vi "Scope Multi Point Read.vi"() -> ()   [LabVIEW 2013]
uses:
  Power Supply.lvlib
  Fixture.lvlib
  Oscilloscope.lvlib
panel:
  in  "outputVoltage":dbl=9.0 format="%#_13g"
  out "Waveform Graph":dbl[](graph)
  in  "Channel":i32=2
  out "error out":errorcluster
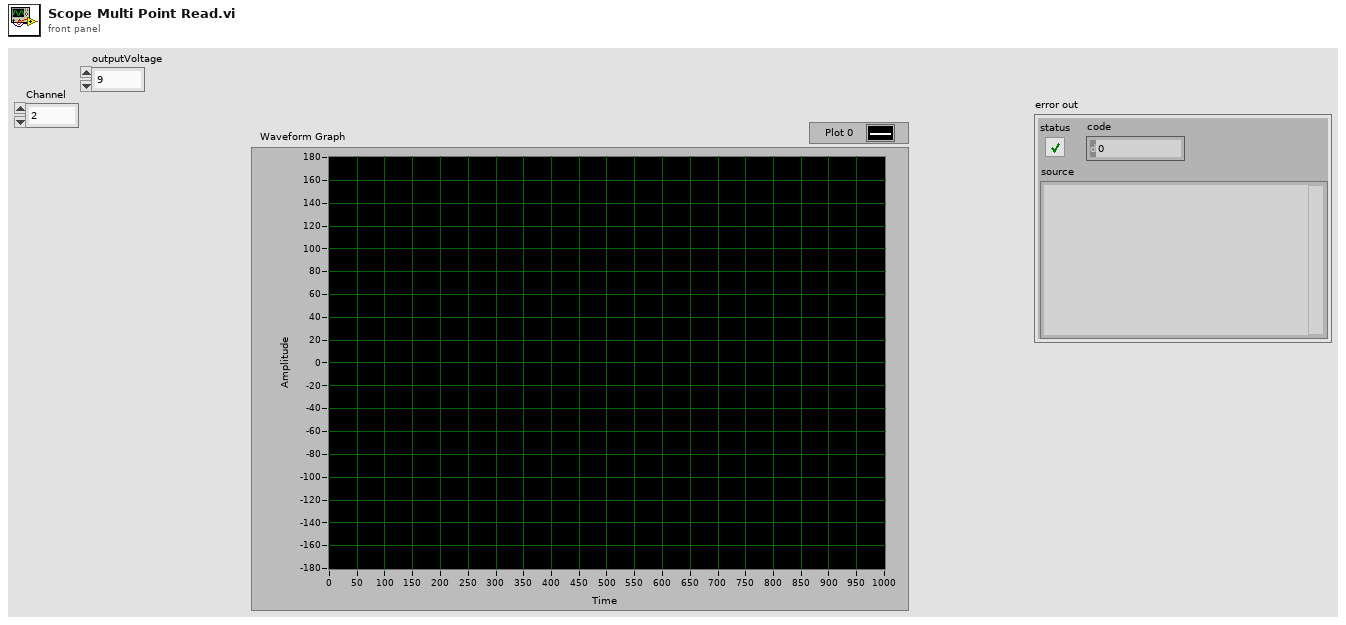
[diagram p1: front panel]
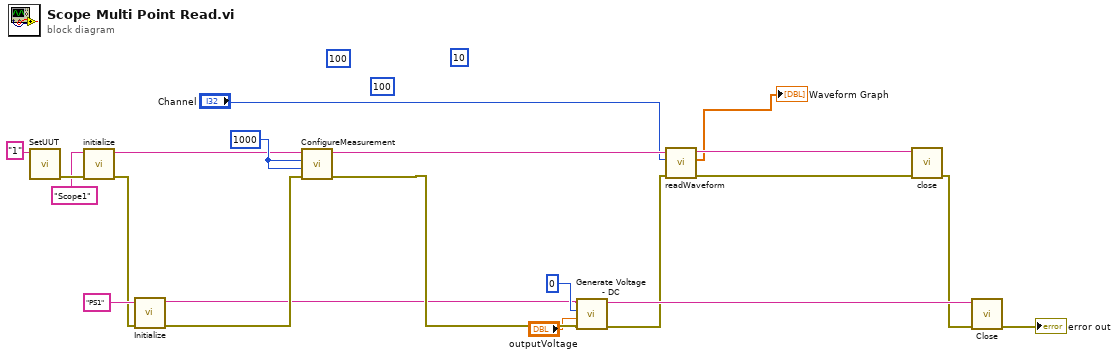
[diagram p0: block diagram]
diagram:
  (unwired) 10
  (unwired) 100
  (unwired) 100
  w10 = 1000 ("numSamples")
  n1 = call "SetUUT.vi"("Serial Number"="1" ("UUTDirectory")) -> ("error out"=w13:errorcluster)  [unwired: 10 in]
  n2 = call "initialize.vi"("error in (no error)"=w13, "Scope in"="Scope1" ("Resource Name")) -> ("error out"=w14:errorcluster, "Scope out"=w9:string)  [unwired: 8 in]
  n3 = call "Initialize.vi"("error in (no error)"=w14, "Power Supply in"="PS1" ("Resource Name")) -> ("error out"=w2:errorcluster, "Power Supply out"=w1:string)  [unwired: 8 in]
  n4 = call "ConfigureMeasurement.vi"("error in (no error)"=w2, "Samples Per Second"=w10, "Number of Samples"=w10, "Scope in"=w9) -> ("error out"=w7:errorcluster, "Scope out"=w11:string)  [unwired: 6 in]
  n5 = call "Generate Voltage - DC.vi"("error in (no error)"=w7, "Output Voltage"="outputVoltage", "Channel"=0 ("channel"), "Power Supply in"=w1) -> ("error out"=w5:errorcluster, "Power Supply out"=w21:string)  [unwired: 6 in]
  n6 = call "readWaveform.vi"("error in (no error)"=w5, "Channel"="Channel", "Scope in"=w11) -> ("error out"=w17:errorcluster, "Result"=→"Waveform Graph":dbl[], "Scope out"=w15:string)  [unwired: 6 in]
  n7 = call "close.vi"("error in (no error)"=w17, "Scope in"=w15) -> ("error out"=w16:errorcluster)  [unwired: 9 in]
  n8 = call "Close.vi"("error in (no error)"=w16, "Power Supply in"=w21) -> ("error out"=→"error out":errorcluster)  [unwired: 9 in]
